vi "BackCellPos.vi"(9 "DisplaySize":T1, 10 "Cell Direction":T2, 11 "Cell Pos":T3) -> (3 "Back Cell Pos":T3)   [LabVIEW 2018, in "Snake.lvclass"]
uses:
  Snake.lvclass
  Typedefs/XYposition.ctl
  Typedefs/UnitDirection.ctl
  Typedefs/DisplaySize.ctl
  BodyCell/SnakeBodyCell.lvclass
panel:
  # "Connector Pane"
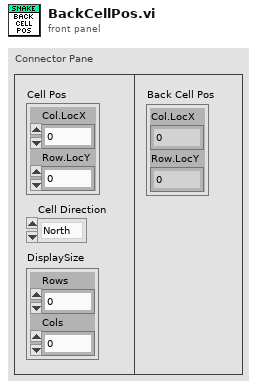
[diagram p1: front panel]
types:
  T1 = typedef "DisplaySize.ctl" = cluster{"Rows":i32, "Cols":i32}
  T2 = typedef "UnitDirection.ctl" = enum16{"North", "East", "South", "West"}
  T3 = typedef "XYposition.ctl" = cluster{"Col.LocX":i32, "Row.LocY":i32}
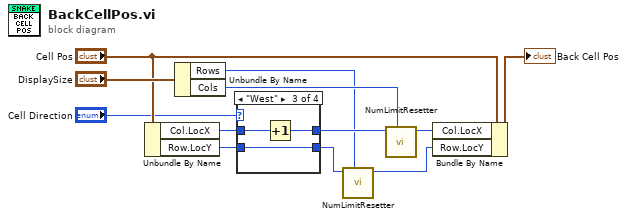
[diagram p0: block diagram]
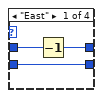
[diagram p2: hidden frame]
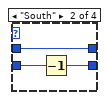
[diagram p3: hidden frame]
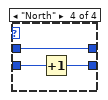
[diagram p4: hidden frame]
diagram:
  n1 = Unbundle By Name("Cell Pos") -> ("Col.LocX"=w10:i32, "Row.LocY"=w9:i32)
  n2 = Unbundle By Name("DisplaySize") -> ("Rows"=w4:i32, "Cols"=w5:i32)
  n3 = case shown="\"West\"" "Cell Direction" {
    tunnel: [w13 w18 w19 w24] -> w12
    tunnel: w10 -> [w15 w18 w21 w24]
    tunnel: [w14 w16 w20 w22] -> w11
    tunnel: w9 -> [w14 w17 w20 w23]
    frame "East" {
      n4 = Decrement(x=w15) -> (x-1=w13:i32)
    }
    frame "South" {
      n5 = Decrement(x=w17) -> (x-1=w16:i32)
    }
    frame "West" {
      n6 = Increment(x=w21) -> (x+1=w19:i32)
    }
    frame "North" {
      n7 = Increment(x=w23) -> (x+1=w22:i32)
    }
  }
  n8 = call "NumLimitResetter.vi"("UpperLimit"=w4, "Num In"=w11) -> ("Num Out"=w7:i32)  [unwired: 9 in]
  n9 = call "NumLimitResetter.vi"("UpperLimit"=w5, "Num In"=w12) -> ("Num Out"=w8:i32)  [unwired: 9 in]
  n10 = Bundle By Name(cluster="Cell Pos", "Col.LocX"=w8, "Row.LocY"=w7) -> (→"Back Cell Pos":T3)
